vi "Wfm wszystkie w lewo.vi"(6 "Position:Left (2)":i32=2, 8 "error in (no error)":errorcluster, 11 "Wfm Refs in":refnum<vi>[](array[refnum])) -> (0 "error out":errorcluster, 3 "Wfm Refs out":refnum<vi>[](array[refnum]))   [LabVIEW 2014]
doc: "Ustawia wszystkie wykresy w jednej osi od lewej strony"
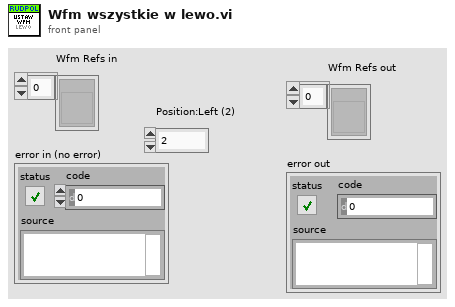
[diagram p1: front panel]
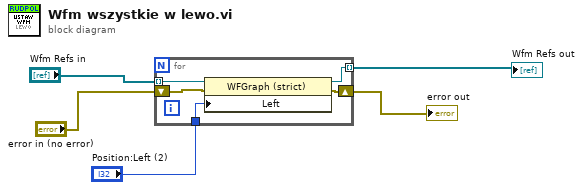
[diagram p0: block diagram]
diagram:
  n1 = for {
    tunnel: "Wfm Refs in" -> [w10] mode=indexing
    tunnel: [w8] -> w4 mode=indexing
    shift-right: [w7] -> w5
    shift-left: "error in (no error)" -> [w9]
    tunnel: "Position:Left (2)" -> [w6]
    n2 = property class="WFGraph (strict)"(reference=w10, error in=w9, "Left"=w6) -> (reference out=w8:refnum<vi>, error out=w7:errorcluster)
  }
  "error out" <- w5
  "Wfm Refs out" <- w4
